vi "Config to String.vi"(8 "error in (no error)":errorcluster, 11 "queue in":T1) -> (0 "error out":errorcluster, 2 "String":string, 3 "queue out":T1)   [LabVIEW 2010, in "NI_LVConfig.lvlib"]
uses:
  NI_LVConfig.lvlib
  Config Queue.ctl
  Config Data.ctl
  Section.ctl
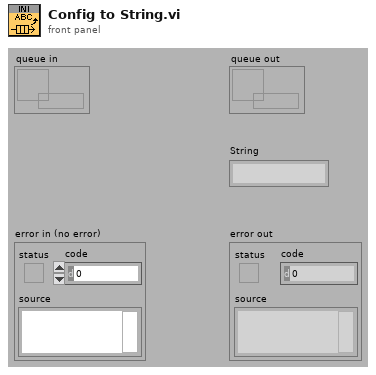
[diagram p1: front panel]
types:
  T1 = typedef "NI_LVConfig.lvlib/Config Queue.ctl" = refnum<queue>
  T2 = typedef "NI_LVConfig.lvlib/Config Data.ctl" = cluster{"sections":T3[], "path":path, "dirty":bool}
  T3 = typedef "NI_LVConfig.lvlib/Section.ctl" = cluster{"name":string, "comment":string, "kvc":string[][]}
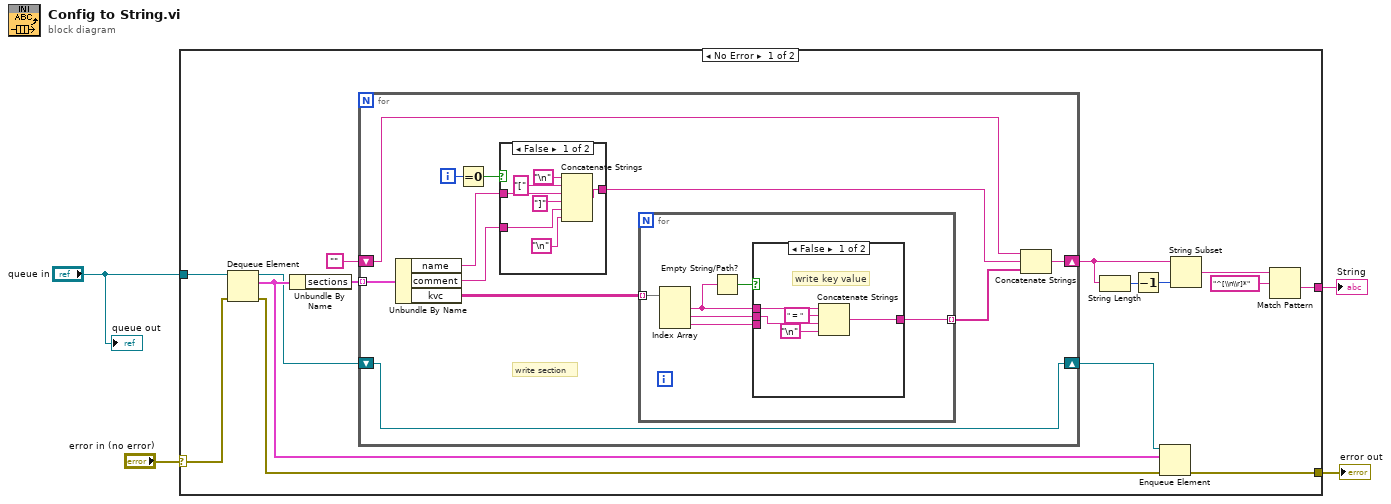
[diagram p0: block diagram]
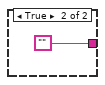
[diagram p2: hidden frame]
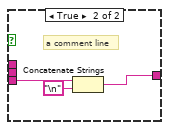
[diagram p3: hidden frame]
diagram:
  n1 = case shown="No Error" "error in (no error)" {
    selector: "error in (no error)" -> [w17 w53]
    tunnel: "queue in" -> [w18 _]
    tunnel: [w14 _] -> w4
    tunnel: [w8 w53] -> w2
    frame No Error {
      n2 = Dequeue Element(queue=w18, error in (no error)=w17) -> (queue out=w6:T1, element=w7:T2, error out=w9:errorcluster)  [unwired: 1 in, 1 out]
      n3 = Unbundle By Name(w7) -> ("sections"=w19:T3[])
      n4 = for {
        tunnel: w19 -> [w30] mode=indexing
        shift-right: [w28] -> w11
        shift-left: "" -> [w27]
        shift-right: [w20] -> w5
        shift-left: w6 -> [w20]
        i -> [w25]
        # "write section"
        n5 = Unbundle By Name(w30) -> ("name"=w26:string, "comment"=w21:string, "kvc"=w22:string[][])
        n6 = Equal To 0?(x=w25) -> (x = 0?=w24:bool)
        n7 = case shown="False" w24 {
          tunnel: w26 -> [w35 _]
          tunnel: [w34 ""] -> w29
          tunnel: w21 -> [w32 _]
          frame False {
            n8 = Concatenate Strings("\n", "[" ("string"), w35, "]" ("string"), w32, "\n") -> (w34:string)
          }
          frame True {
          }
        }
        n9 = for {
          tunnel: w22 -> [w44] mode=indexing
          tunnel: [w41] -> w23 mode=indexing
          n10 = Index Array(array=w44) -> (element #1=w39:string, element #2=w40:string, element #3=w42:string)  [unwired: 3 in]
          n11 = Empty String/Path?(string/path=w39) -> (empty?=w43:bool)
          n12 = case shown="False" w43 {
            tunnel: w42 -> [_ w52]
            tunnel: [w45 w50] -> w41
            tunnel: w40 -> [w47 _]
            tunnel: w39 -> [w49 _]
            frame False {
              # "write key value"
              n13 = Concatenate Strings(w49, " = " ("string"), w47, "\n") -> (w45:string)
            }
            frame True {
              # "a comment line"
              n14 = Concatenate Strings(w52, "\n") -> (w50:string)
            }
          }
        }
        n15 = Concatenate Strings(w27, w29, w23) -> (w28:string)
      }
      n16 = String Length(string=w11) -> (length=w13:i32)
      n17 = Decrement(x=w13) -> (x-1=w12:i32)
      n18 = Enqueue Element(queue=w5, element=w7, error in (no error)=w9) -> (error out=w8:errorcluster)  [unwired: 1 in, 2 out]
      n19 = String Subset(string=w11, length (rest)=w12) -> (substring=w10:string)  [unwired: 1 in]
      n20 = Match Pattern(string=w10, regular expression="^[\\n\\r]*") -> (after substring=w14:string)  [unwired: 1 in, 3 out]
    }
    frame Error {
    }
  }
  "error out" <- w2
  "String" <- w4
  "queue out" <- "queue in"
